vi "Get or Create Master Reference.vi"(8 "error in":errorcluster, 11 "Main VI Path":path) -> (0 "error out":errorcluster, 2 "New Reference Created":bool, 3 "Master Reference":T1)   [LabVIEW 2023, in "EL72xx_DMC_ServoAxis.lvlib" / "VI Reference Management.lvlib"]
doc: "Returns the master VI reference for the cloneable Main VI. If that reference has not been created yet, this VI creates it and lets the caller know.\n_____\nBased on DQMH Project Template 7.0.1.1316."
uses:
  VI Reference Management.lvlib
  Main VI Type--strict_vi_ref.ctl
  <vilib>/Delacor/Delacor QMH/Libraries/Cloneable Module Admin_class/Delacor_lib_QMH_Cloneable Module Admin.lvclass
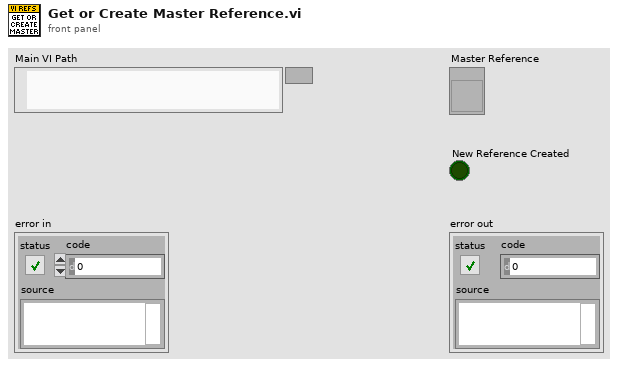
[diagram p1: front panel]
types:
  T1 = typedef "EL72xx_DMC_ServoAxis.lvlib/VI Reference Management.lvlib/Main VI Type--strict_vi_ref.ctl" = refnum<vi>
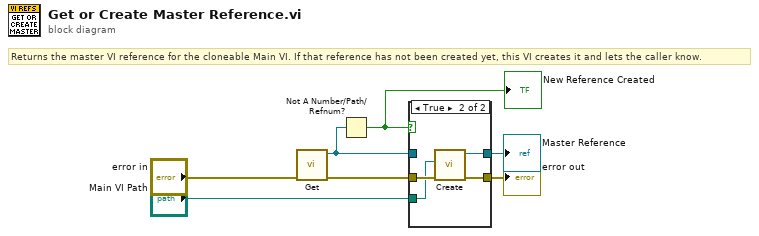
[diagram p0: block diagram]
diagram:
  # "Returns the master VI reference for the cloneable Main VI. If that reference has not been created yet, this VI creates it and lets the caller know."
  n1 = call "Get.vi"("error in"="error in") -> ("error out"=w6:errorcluster, "Master Reference"=w5:T1)  [unwired: 9 in]
  n2 = Not A Number/Path/Refnum?(number/path/refnum=w5) -> (NaN/Path/Refnum?=w2:bool)
  "New Reference Created" <- w2
  n3 = case shown="True" w2 {
    tunnel: w6 -> [w8 w13]
    tunnel: w5 -> [w9 _]
    tunnel: [w9 w11] -> w4
    tunnel: [w8 w12] -> w3
    tunnel: "Main VI Path" -> [_ w10]
    frame False {
    }
    frame True {
      n4 = call "Create.vi"("error in"=w13, "Main VI Path"=w10) -> ("error out"=w12:errorcluster, "Master Reference"=w11:T1)  [unwired: 8 in]
    }
  }
  "Master Reference" <- w4
  "error out" <- w3
